vi "Read.vi"(8 "error in (no error)":errorcluster, 11 "Test Type A in":refnum<class "Test Type A.lvclass">) -> (0 "error out":errorcluster, 2 "Value":string, 3 "Test Type A out":refnum<class "Test Type A.lvclass">)   [LabVIEW 2020, in "Test Type A.lvclass"]
uses:
  Test Type A.lvclass
  Test Type A.lvclass/Test Type A.ctl
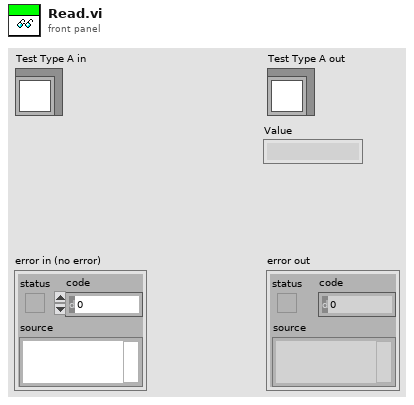
[diagram p1: front panel]
types:
  T1 = typedef "Test Type A.lvclass/Ref Data.ctl" = cluster{"Value":string}
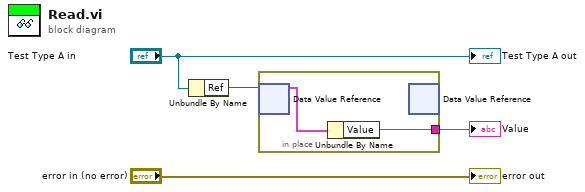
[diagram p0: block diagram]
diagram:
  n1 = Unbundle By Name("Test Type A in") -> ("Ref"=w3:refnum<data-value>)
  n2 = in-place {
    in-place-border: [w5] -> w1
    n3 = in-place-dvr #1(w3) -> (w6:T1)  [unwired: 1 out]
    n4 = Unbundle By Name(w6) -> ("Value"=w5:string)
    n5 = in-place-dvr #1() -> ()  [unwired: 1 in, 2 out]
  }
  "Value" <- w1
  "error out" <- "error in (no error)"
  "Test Type A out" <- "Test Type A in"
